vi "add_element(array).vi"(8 "error in (no error)":errorcluster, 10 "element":cluster{"name":string, "address":string}, 11 "data store (in)":cluster{"name":string, "address":string}[](array[cluster])) -> (0 "error out":errorcluster, 3 "data store (out)":cluster{"name":string, "address":string}[](array[cluster]))   [LabVIEW 2018]
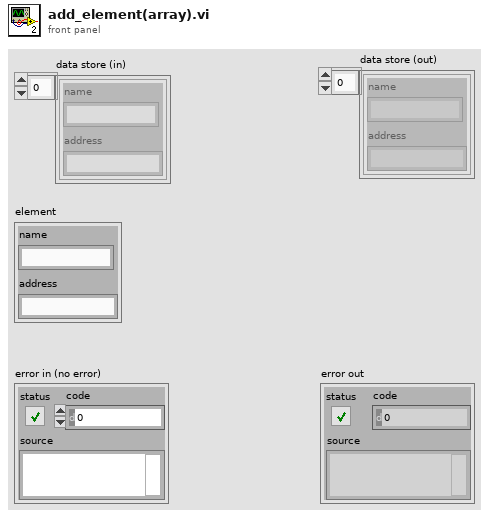
[diagram p1: front panel]
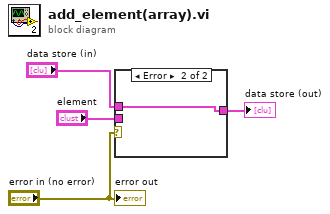
[diagram p0: block diagram]
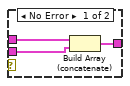
[diagram p2: hidden frame]
diagram:
  n1 = case shown="Error" "error in (no error)" {
    tunnel: "data store (in)" -> [w7 w8]
    tunnel: "element" -> [w6 _]
    tunnel: [w5 w8] -> w2
    frame No Error {
      n2 = Build Array (concatenate)(w7, w6) -> (w5:cluster{"name":string, "address":string}[])
    }
    frame Error {
    }
  }
  "data store (out)" <- w2
  "error out" <- "error in (no error)"
